vi "Edycja_blokuj_kursory.vi"(8 "error in (no error)":errorcluster, 10 "Zablokowane free in":T1[](array[typedef]), 11 "Wykres Ref":refnum<vi>) -> (0 "error out":errorcluster, 2 "Zablokowane free out":T1[](array[typedef]))   [LabVIEW 2014]
doc: "Realizuje blokowanie kursorów swobodnych,\njeśli taką opcję zaznaczono"
uses:
  Kontrolki/GUI/Edycja_blokowanie_free.ctl
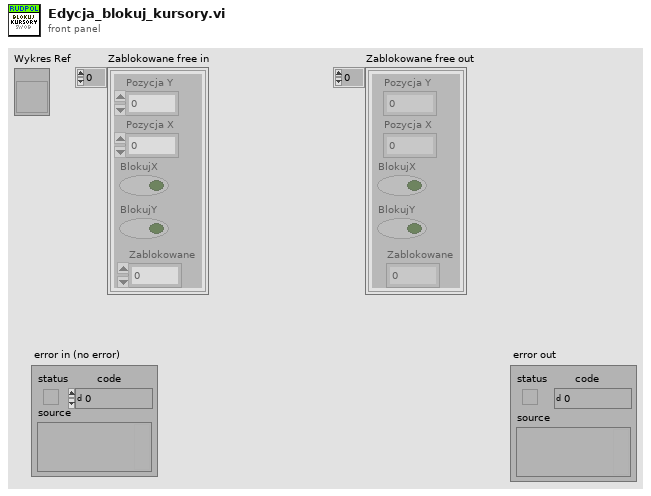
[diagram p1: front panel]
types:
  T1 = typedef "Edycja_blokowanie_free.ctl" = cluster{"Pozycja Y":dbl, "Pozycja X":dbl, "BlokujX":bool, "BlokujY":bool, "Zablokowane":i32}
  T2 = typedef "LVCursorListTypeDef.ctl" = cluster{"Name":string, "Color":u32, "Style":u8, "Point Style":u8, "Name Visible":bool, "Allow Drag":bool, "Cursor Mode":u32, "Plot":i32, "Index":i32, "Position":cluster{"X":dbl, "Y":dbl}, "X Scale":u32, "Y Scale":u32, "Watch Plots":i32[], "Watch All Plots":bool, "Plot Area":i32, "Label Offset":cluster{"X":dbl, "Y":dbl}}[]
  T3 = cluster{"Name":string, "Color":u32, "Style":u8, "Point Style":u8, "Name Visible":bool, "Allow Drag":bool, "Cursor Mode":u32, "Plot":i32, "Index":i32, "Position":cluster{"X":dbl, "Y":dbl}, "X Scale":u32, "Y Scale":u32, "Watch Plots":i32[], "Watch All Plots":bool, "Plot Area":i32, "Label Offset":cluster{"X":dbl, "Y":dbl}}
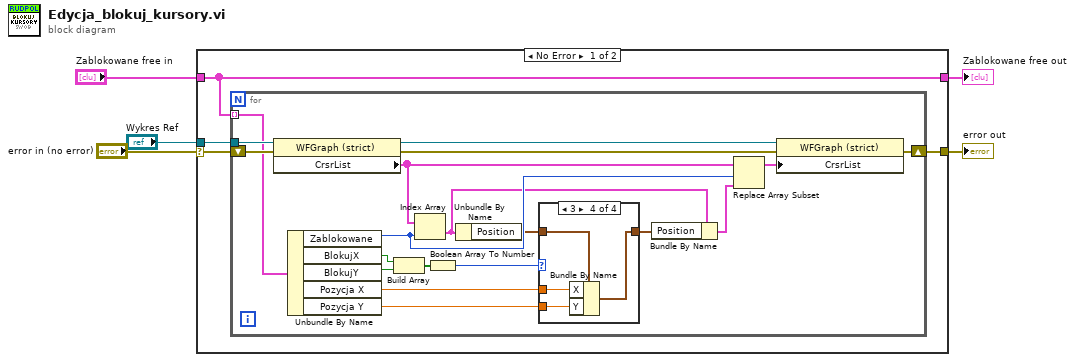
[diagram p0: block diagram]
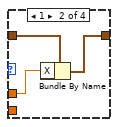
[diagram p3: hidden frame]
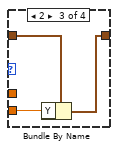
[diagram p4: hidden frame]
diagram:
  n1 = case shown="No Error" "error in (no error)" {
    selector: "error in (no error)" -> [w7 w41]
    tunnel: [w6 w41] -> w4
    tunnel: "Wykres Ref" -> [w8 _]
    tunnel: "Zablokowane free in" -> [w9 w40]
    tunnel: [w9 w40] -> w1
    frame No Error {
      n2 = for {
        tunnel: w9 -> [w23] mode=indexing
        tunnel: w8 -> [w28]
        shift-right: [w24] -> w6
        shift-left: w7 -> [w27]
        n3 = property class="WFGraph (strict)"(reference=w28, error in=w27) -> (reference out=w26:refnum<vi>, error out=w25:errorcluster, "CrsrList"=w21:T2)
        n4 = Unbundle By Name(w23) -> ("Zablokowane"=w22:i32, "BlokujX"=w19:bool, "BlokujY"=w18:bool, "Pozycja X"=w14:dbl, "Pozycja Y"=w10:dbl)
        n5 = Build Array(w19, w18) -> (w17:bool[])
        n6 = Index Array(array=w21, index=w22) -> (element=w13:T3)
        n7 = Boolean Array To Number(Boolean array=w17) -> (number=w16:u32)
        n8 = Unbundle By Name(w13) -> ("Position"=w15:cluster{"X":dbl, "Y":dbl})
        n9 = case shown="3" w16 {
          tunnel: w15 -> [w29 w32 w35 w39]
          tunnel: w14 -> [_ w31 _ w38]
          tunnel: [w29 w30 w34 w36] -> w12
          tunnel: w10 -> [_ _ w33 w37]
          frame 0, Default {
          }
          frame 1 {
            n10 = Bundle By Name(cluster=w32, "X"=w31) -> (w30:cluster{"X":dbl, "Y":dbl})
          }
          frame 2 {
            n11 = Bundle By Name(cluster=w35, "Y"=w33) -> (w34:cluster{"X":dbl, "Y":dbl})
          }
          frame 3 {
            n12 = Bundle By Name(cluster=w39, "X"=w38, "Y"=w37) -> (w36:cluster{"X":dbl, "Y":dbl})
          }
        }
        n13 = Bundle By Name(cluster=w13, "Position"=w12) -> (w11:T3)
        n14 = Replace Array Subset(array=w21, new element=w11, index=w22) -> (w20:T2)
        n15 = property class="WFGraph (strict)"(reference=w26, error in=w25, "CrsrList"=w20) -> (error out=w24:errorcluster)  [unwired: 1 out]
      }
    }
    frame Error {
    }
  }
  "error out" <- w4
  "Zablokowane free out" <- w1
